vi "Disconnect.vi"(8 "error in (no error)":errorcluster, 11 "B&K Precision 9120 series in":refnum<class "B&K Precision 9120 series.lvclass">) -> (0 "error out":errorcluster)   [LabVIEW 2014, in "B&K Precision 9120 series.lvclass"]
uses:
  B&K Precision 9120 series.lvclass
  B&K Precision 9120 series.lvclass/B&K Precision 9120 series.ctl
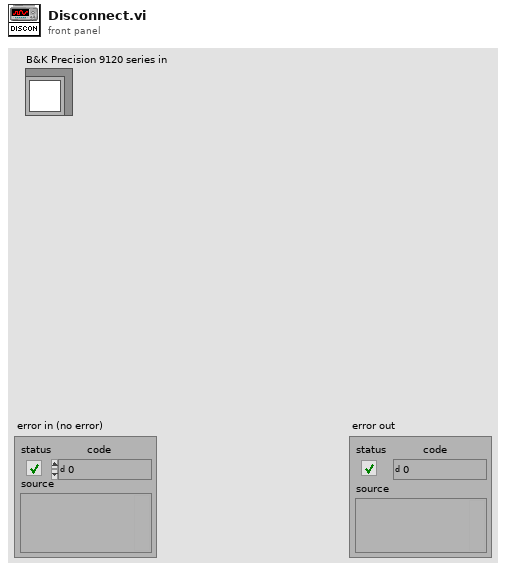
[diagram p1: front panel]
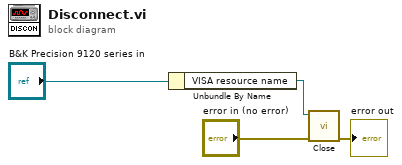
[diagram p0: block diagram]
diagram:
  n1 = Unbundle By Name("B&K Precision 9120 series in") -> ("VISA resource name"=w1:refnum<visa-resource-name>)
  n2 = call "Close.vi"("error in (no error)"="error in (no error)", "VISA resource in"=w1) -> ("error out"=→"error out":errorcluster)  [unwired: 9 in]
